vi "Log Write.vi"(4 "Write Header":bool, 8 "Measurement In":refnum<data-value>, 9 "State Estimate In":refnum<data-value>, 10 "Log Handle In":T1, 11 "Error In":errorcluster) -> (0 "Measurement Out":refnum<data-value>, 1 "State Estimate Out":refnum<data-value>, 2 "Log Handle Out":T1, 3 "Error Out":errorcluster, 5 "Logged Events":string[](array[string]))   [LabVIEW 2019]
uses:
  State Estimator/Measurements.ctl
  IMU/IMU Data.ctl
  Steering Motor Encoder/Steering Motor Encoder Data.ctl
  GNSS/GNSS Data.ctl
  State Estimator/State Estimate.ctl
  Log Handle.ctl
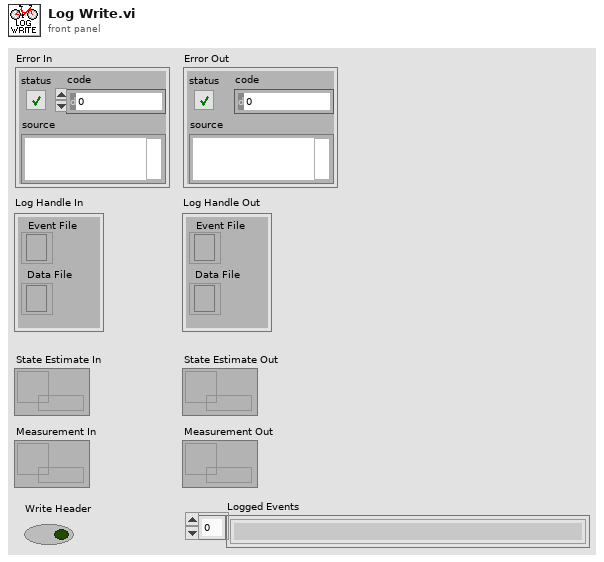
[diagram p1: front panel]
types:
  T1 = typedef "Log Handle.ctl" = cluster{"Data File":refnum<file>, "Event File":refnum<file>}
  T2 = typedef "State Estimate.ctl" = cluster{"X (m)":dbl, "Y (m)":dbl, "Psi (rad)":dbl, "Roll (rad)":dbl, "Roll Rate (rad/s)":dbl}
  T3 = typedef "Measurements.ctl" = cluster{"IMU Data":T4, "Steering Motor Encoder Data":T5, "GNSS Data":T6}
  T4 = typedef "IMU Data.ctl" = cluster{"Gyroscope":cluster{"X (rad/s)":dbl, "Y (rad/s)":dbl, "Z (rad/s)":dbl}, "Accelerometer":cluster{"X (m/s^2)":dbl, "Y (m/s^2)":dbl, "Z (m/s^2)":dbl}}
  T5 = typedef "Steering Motor Encoder Data.ctl" = cluster{"Encoder Position (counts)":i32, "Steering Angle (rad)":dbl}
  T6 = typedef "GNSS Data.ctl" = cluster{"Latitude (rad)":dbl, "Longitude (rad)":dbl, "Altitude (m)":dbl, "Speed (m/s)":dbl, "Heading (rad)":dbl, "Fix Quality":i32, "Number of Satellites":i32, "Latitude (deg)":dbl, "Longitude (deg)":dbl}
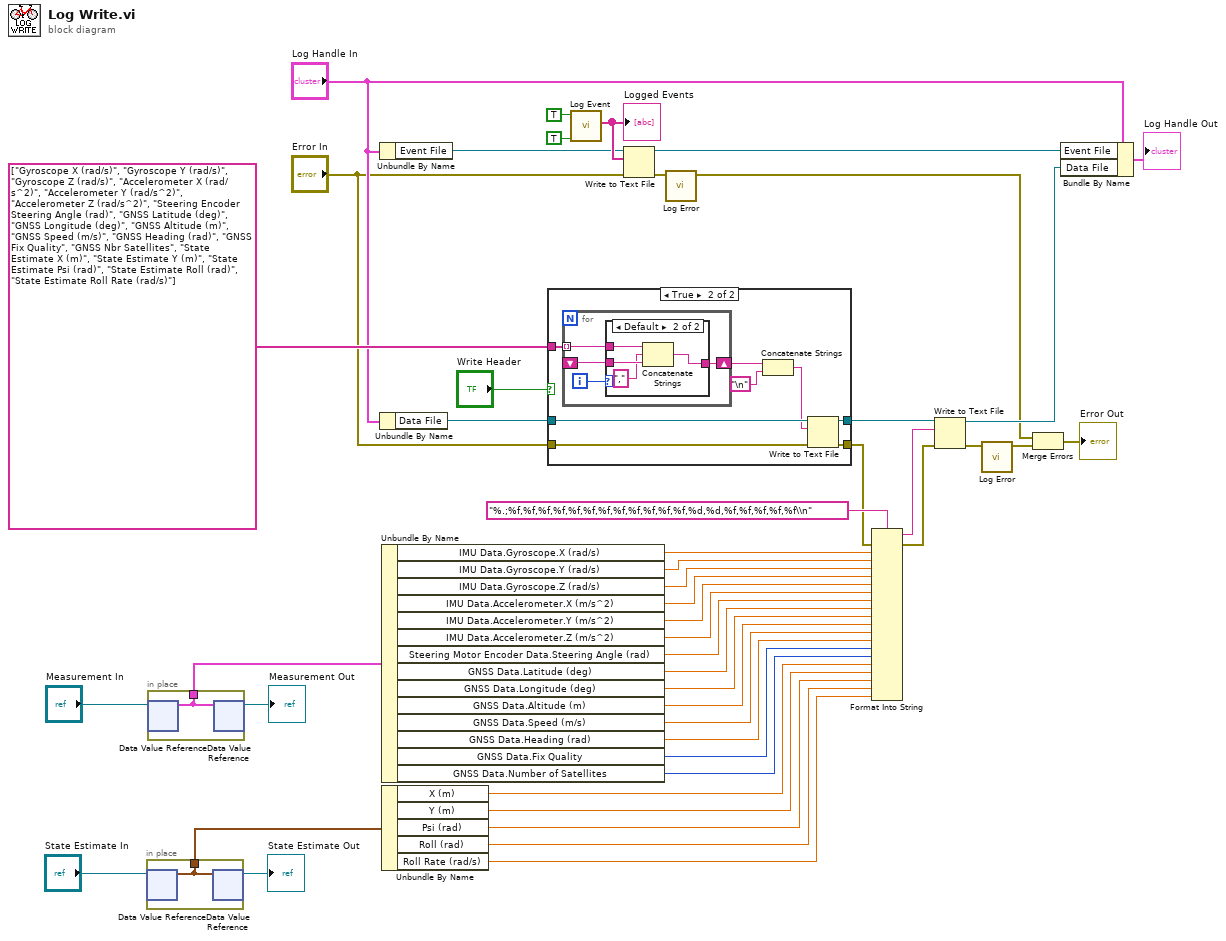
[diagram p0: block diagram]
diagram:
  n1 = in-place {
    in-place-border: [w48] -> w42
    n2 = in-place-dvr #1("State Estimate In") -> (w48:T2)  [unwired: 1 out]
    n3 = in-place-dvr #1(w48) -> (→"State Estimate Out":refnum<data-value>)  [unwired: 1 out]
  }
  n4 = in-place {
    in-place-border: [w49] -> w43
    n5 = in-place-dvr #2("Measurement In") -> (w49:T3)  [unwired: 1 out]
    n6 = in-place-dvr #2(w49) -> (→"Measurement Out":refnum<data-value>)  [unwired: 1 out]
  }
  n7 = Unbundle By Name("Log Handle In") -> ("Event File"=w10:refnum<file>)
  n8 = Unbundle By Name("Log Handle In") -> ("Data File"=w40:refnum<file>)
  n9 = Unbundle By Name(w43) -> ("IMU Data.Gyroscope.X (rad/s)"=w38:dbl, "IMU Data.Gyroscope.Y (rad/s)"=w37:dbl, "IMU Data.Gyroscope.Z (rad/s)"=w36:dbl, "IMU Data.Accelerometer.X (m/s^2)"=w35:dbl, "IMU Data.Accelerometer.Y (m/s^2)"=w34:dbl, "IMU Data.Accelerometer.Z (m/s^2)"=w33:dbl, "Steering Motor Encoder Data.Steering Angle (rad)"=w32:dbl, "GNSS Data.Latitude (deg)"=w31:dbl, "GNSS Data.Longitude (deg)"=w30:dbl, "GNSS Data.Altitude (m)"=w29:dbl, "GNSS Data.Speed (m/s)"=w28:dbl, "GNSS Data.Heading (rad)"=w27:dbl, "GNSS Data.Fix Quality"=w26:i32, "GNSS Data.Number of Satellites"=w25:i32)
  n10 = Unbundle By Name(w42) -> ("X (m)"=w23:dbl, "Y (m)"=w22:dbl, "Psi (rad)"=w21:dbl, "Roll (rad)"=w20:dbl, "Roll Rate (rad/s)"=w19:dbl)
  n11 = case shown="True" "Write Header" {
    tunnel: string[] ["Gyroscope X (rad/s)", "Gyroscope Y (rad/s)", "Gyroscope Z (rad/s)", "Accelerometer X (rad/s^2)", "Accelerometer Y (rad/s^2)", "Accelerometer Z (rad/s^2)", "Steering Encoder Steering Angle (rad)", "GNSS Latitude (deg)", "GNSS Longitude (deg)", "GNSS Altitude (m)", "GNSS Speed (m/s)", "GNSS Heading (rad)", "GNSS Fix Quality", "GNSS Nbr Satellites", "State Estimate X (m)", "State Estimate Y (m)", "State Estimate Psi (rad)", "State Estimate Roll (rad)", "State Estimate Roll Rate (rad/s)"] ("channel name(s) in (Untitled)") -> [_ w59]
    tunnel: w40 -> [w51 w58]
    tunnel: "Error In" -> [w50 w57]
    tunnel: [w51 w56] -> w18
    tunnel: [w50 w55] -> w16
    frame False {
    }
    frame True {
      n12 = for {
        tunnel: w59 -> [w63] mode=indexing
        shift-right: [w61] -> w54
        shift-left: _ -> [w60]
        i -> [w62]
        n13 = case shown="Default" w62 {
          tunnel: w63 -> [w64 w68]
          tunnel: [w64 w67] -> w61
          tunnel: w60 -> [_ w66]
          frame 0 {
          }
          frame Default {
            n14 = Concatenate Strings(w68, "," ("string"), w66) -> (w67:string)
          }
        }
      }
      n15 = Concatenate Strings(w54, "\n") -> (w53:string)
      n16 = Write to Text File(file (use dialog)=w58, text=w53, error in=w57) -> (refnum out=w56:refnum<file>, error out=w55:errorcluster)  [unwired: 1 in, 1 out]
    }
  }
  n17 = call "Log Event.vi"("Clear Log"=TRUE, "Read"=TRUE) -> ("All Events"=w12:string[])  [unwired: 9 in]
  "Logged Events" <- w12
  n18 = Write to Text File(file (use dialog)=w10, text=w12, error in="Error In") -> (refnum out=w7:refnum<file>, error out=w6:errorcluster)  [unwired: 1 in, 1 out]
  n19 = call "Log Error.vi"("Error In"=w6) -> ("Error Out"=w3:errorcluster)  [unwired: 10 in]
  n20 = Format Into String(format string="%.;%f,%f,%f,%f,%f,%f,%f,%f,%f,%f,%f,%f,%d,%d,%f,%f,%f,%f,%f\\n", error in=w16, w38, w37, w36, w35, w34, w33, w32, w31, w30, w29, w28, w27, w26, w25, w23, w22, w21, w20, w19) -> (resulting string=w17:string, error out=w15:errorcluster)  [unwired: 1 in]
  n21 = Write to Text File(file (use dialog)=w18, text=w17, error in=w15) -> (refnum out=w8:refnum<file>, error out=w5:errorcluster)  [unwired: 1 in, 1 out]
  n22 = call "Log Error.vi"("Error In"=w5) -> ("Error Out"=w4:errorcluster)  [unwired: 10 in]
  n23 = Merge Errors(w3, w4) -> (→"Error Out":errorcluster)
  n24 = Bundle By Name(cluster="Log Handle In", "Event File"=w7, "Data File"=w8) -> (→"Log Handle Out":T1)
